vi "zad2.vi"() -> ()   [LabVIEW 2018]
doc: "Use this template to build a producer/consumer design pattern with events to produce queue items. Use this design pattern instead of the User Interface Event Handler pattern for user interfaces when you want to execute code asynchronously in response to an event without slowing the user interface responsiveness."
panel:
  out "Action 2":bool
  out "Action 1":bool
  in  "Action 2":bool
  in  "Action1":bool
  in  "stop":bool
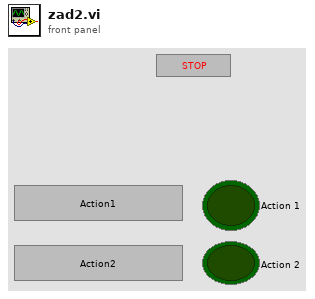
[diagram p1: front panel]
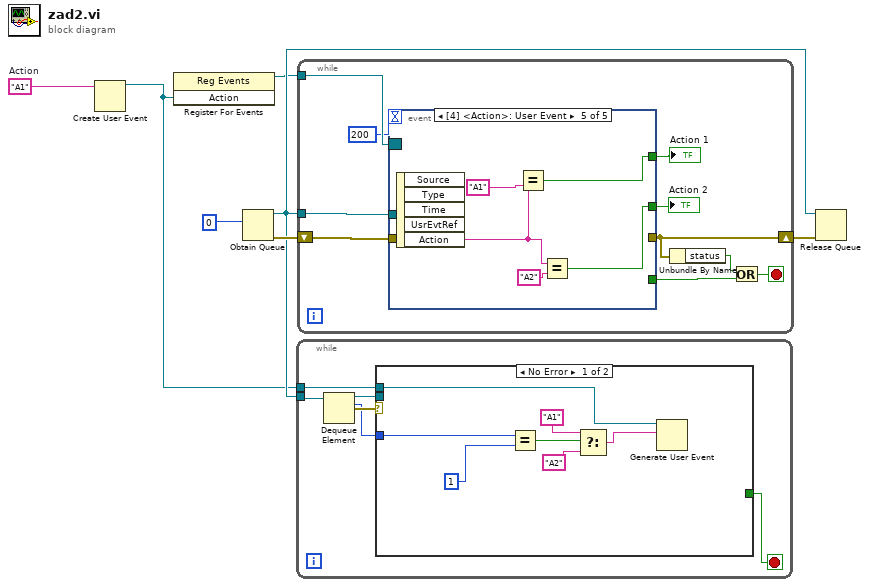
[diagram p0: block diagram]
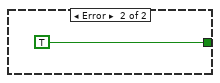
[diagram p2: hidden frame]
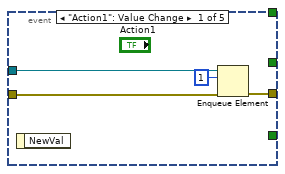
[diagram p3: hidden frame]
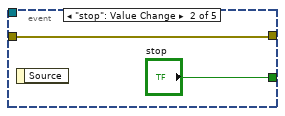
[diagram p4: hidden frame]
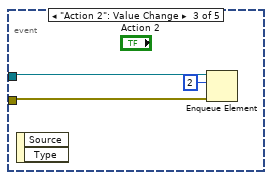
[diagram p5: hidden frame]
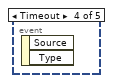
[diagram p6: hidden frame]
diagram:
  w3 = "A1"  # Action
  n1 = Create User Event(user event datatype=w3) -> (user event=w1:refnum<user-event>)  [unwired: 1 in, 1 out]
  n2 = register-events(w1) -> (reference out=w2:refnum<event-registration>)  [unwired: 2 in, 1 out]
  n3 = Obtain Queue(element data type=0) -> (queue out=w5:refnum<queue>, error out=w7:errorcluster)  [unwired: 4 in, 1 out]
  n4 = while {
    tunnel: w5 -> [w13]
    tunnel: w1 -> [w8]
    stop <- w11 stop-if-true
    n5 = Dequeue Element(queue=w13) -> (queue out=w10:refnum<queue>, element=w9:i32, error out=w12:errorcluster)  [unwired: 2 in, 1 out]
    n6 = case shown="No Error" w12 {
      tunnel: [_ TRUE] -> w11
      tunnel: w10 -> [_ _]
      tunnel: w9 -> [w20 _]
      tunnel: w8 -> [w15 _]
      frame No Error {
        n7 = Equal?(x=w20, y=1 ("element")) -> (x = y?=w18:bool)
        n8 = Select(t="A1", s=w18, f="A2") -> (s? t:f=w14:string)
        n9 = Generate User Event(user event=w15, event data cluster=w14) -> ()  [unwired: 2 in, 2 out]
      }
      frame Error {
      }
    }
  }
  n10 = while {
    shift-right: [w27] -> w6
    shift-left: w7 -> [w30]
    tunnel: w5 -> [w31]
    tunnel: w2 -> [w23]
    stop <- w28 stop-if-true
    n11 = event shown="[4] <Action>: User Event" {
      selector: w23 -> [_ _ _ _ _]
      dyn-events: _ -> [_ _ _ _ _]
      timeout: u32 200 ("milliseconds to wait") -> [_ _ _ _ _]
      tunnel: w31 -> [w35 _ w40 _ _]
      tunnel: w30 -> [w34 w36 w39 _ _]
      tunnel: [w33 w36 _ _ _] -> w27
      tunnel: [_ "stop" _ _ _] -> w29
      tunnel: [_ _ _ _ w45] -> w25
      tunnel: [_ _ _ _ w42] -> w24
      event "Action1": Value Change {
        n12 = event-data() -> ()  [unwired: 1 in, 1 out]
        n13 = Enqueue Element(queue=w35, element=1, error in (no error)=w34) -> (error out=w33:errorcluster)  [unwired: 1 in, 2 out]
      }
      event "stop": Value Change {
        n14 = event-data() -> ()  [unwired: 1 in, 1 out]
      }
      event "Action 2": Value Change {
        n15 = event-data() -> ()  [unwired: 1 in, 2 out]
        n16 = Enqueue Element(queue=w40, element=2, error in (no error)=w39) -> ()  [unwired: 1 in, 3 out]
      }
      event Timeout {
        n17 = event-data() -> ()  [unwired: 1 in, 2 out]
      }
      event User Event {
        n18 = event-data() -> ("Action"=w43:string)  [unwired: 1 in, 4 out]
        n19 = Equal?(x=w43, y="A1") -> (x = y?=w45:bool)
        n20 = Equal?(x=w43, y="A2" ("f")) -> (x = y?=w42:bool)
      }
    }
    "Action 1" <- w25
    "Action 2" <- w24
    n21 = Unbundle By Name(w27) -> ("status"=w26:bool)
    n22 = Or(x=w26, y=w29) -> (x .or. y?=w28:bool)
  }
  n23 = Release Queue(queue=w5, error in (no error)=w6) -> ()  [unwired: 1 in, 3 out]
